vi "RenameFiles.vi"() -> ()   [LabVIEW 2022 SP3]
panel:
  out "filenames":string[](array[string])
  in  "directory path of data and header file":path
  in  "search pattern":string="*VPI.raw"
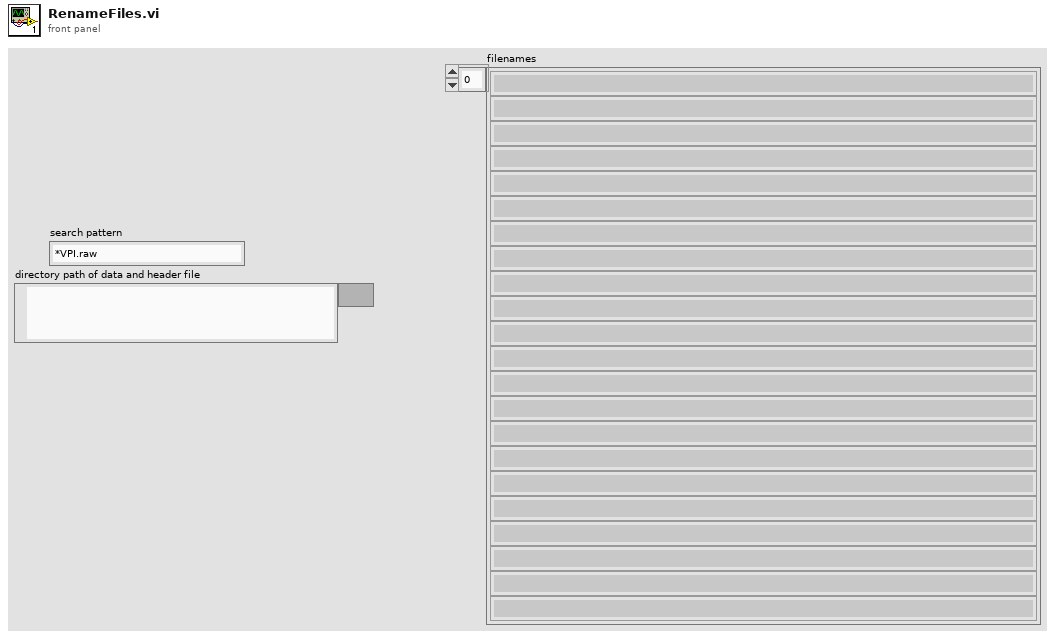
[diagram p1: front panel]
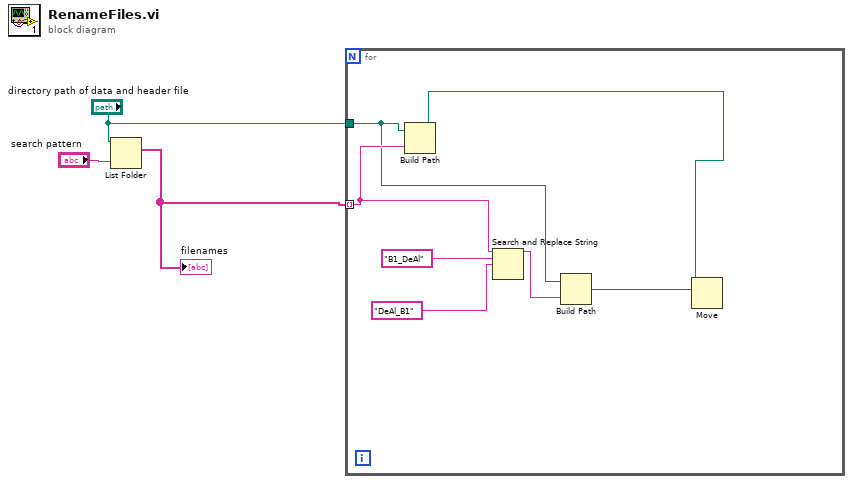
[diagram p0: block diagram]
diagram:
  n1 = List Folder(path="directory path of data and header file", pattern="search pattern") -> (filenames=w2:string[])  [unwired: 1 in, 4 out]
  "filenames" <- w2
  n2 = for {
    tunnel: w2 -> [w10] mode=indexing
    tunnel: "directory path of data and header file" -> [w7]
    n3 = Build Path(base path=w7, name or relative path=w10) -> (appended path=w4:path)
    n4 = Search and Replace String(input string=w10, search string="B1_DeAl", replace string="DeAl_B1") -> (result string=w6:string)  [unwired: 5 in, 3 out]
    n5 = Build Path(base path=w7, name or relative path=w6) -> (appended path=w5:path)
    n6 = Move(source path=w4, 10:w5) -> ()  [unwired: 3 in, 3 out]
  }
